vi "Sub_Preprocessing_Main.vi"(11 "Experiment in":T1) -> (3 "Experiment out":T1)   [LabVIEW 2021]
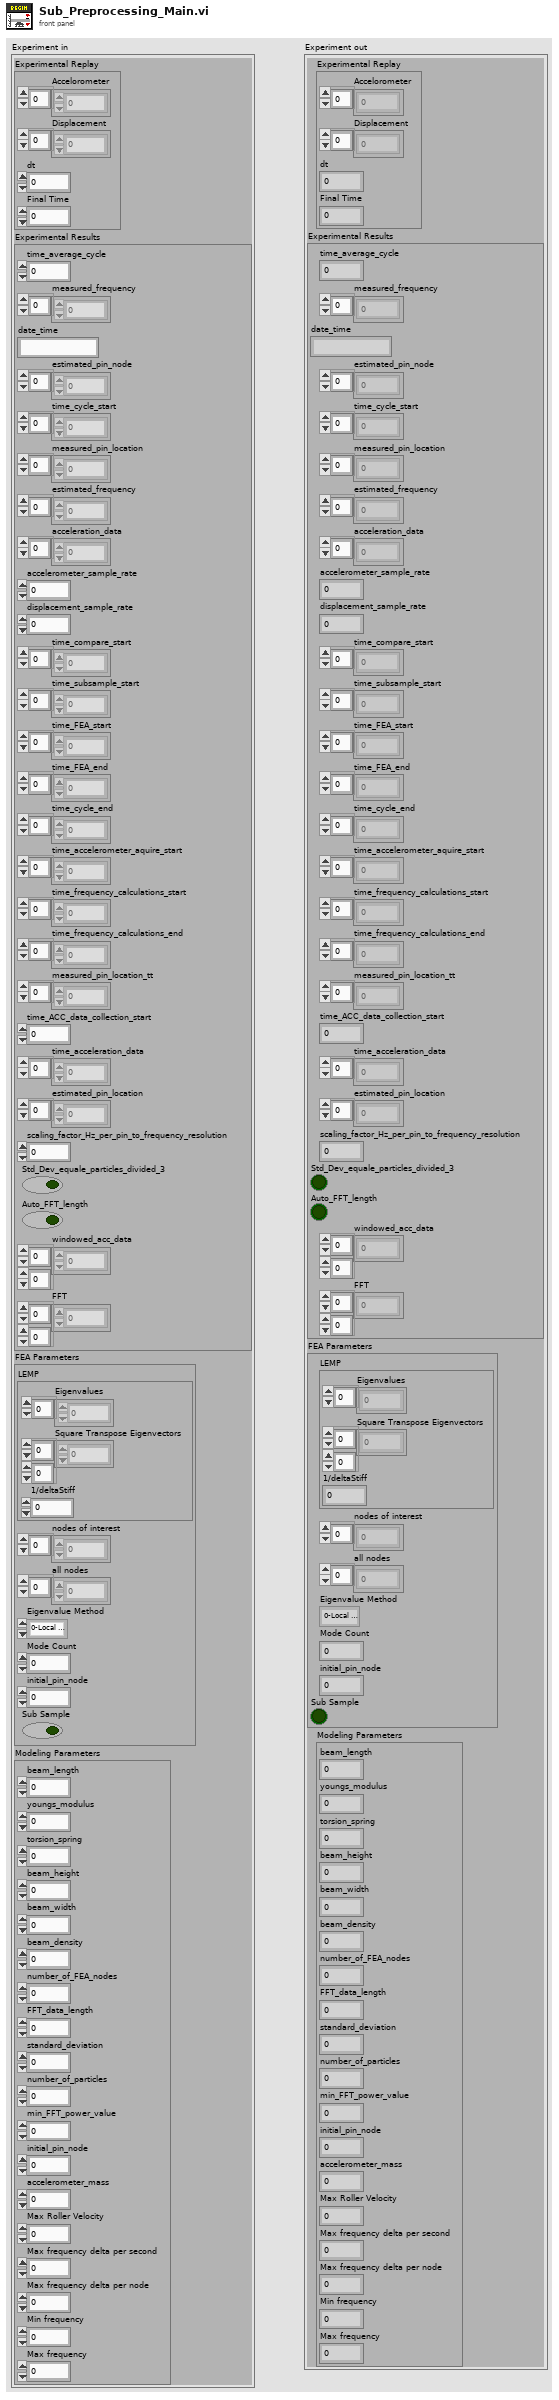
[diagram p1: front panel]
types:
  T1 = cluster{"Experimental Replay":cluster{"Accelorometer":dbl[], "Displacement":dbl[], "dt":dbl, "Final Time":dbl}, "Experimental Results":cluster{"time_average_cycle":dbl, "measured_frequency":dbl[], "date_time":string, "estimated_pin_node":i32[], "time_cycle_start":dbl[], "measured_pin_location":dbl[], "estimated_frequency":dbl[], "acceleration_data":dbl[], "accelerometer_sample_rate":dbl, "displacement_sample_rate":dbl, "time_compare_start":dbl[], "time_subsample_start":dbl[], "time_FEA_start":dbl[], "time_FEA_end":dbl[], "time_cycle_end":dbl[], "time_accelerometer_aquire_start":dbl[], "time_frequency_calculations_start":dbl[], "time_frequency_calculations_end":dbl[], "measured_pin_location_tt":dbl[], "time_ACC_data_collection_start":dbl, "time_acceleration_data":dbl[], "estimated_pin_location":dbl[], "scaling_factor_Hz_per_pin_to_frequency_resolution":dbl, "Std_Dev_equale_particles_divided_3":bool, "Auto_FFT_length":bool, "windowed_acc_data":dbl[][], "FFT":dbl[][]}, "FEA Parameters":cluster{"LEMP":cluster{"Eigenvalues":dbl[], "Square Transpose Eigenvectors":dbl[][], "1/deltaStiff":dbl}, "nodes of interest":i32[], "all nodes":i32[], "Eigenvalue Method":enum16{"0-Local Eigen Modification Procedure", "1-LabVIEW generalized eigenvalues", "2-LabVIEW M^-1K eigenvalues", "3-LabVIEW Cholesky Factorization", "4-Cholesky Factorization CPU SGL", "5-Cholesky Factorization CPU FXP", "6-Cholesky Factorization FPGA SGL", "7-Cholesky Factorization FPGA SGL SCL"}, "Mode Count":i32, "initial_pin_node":i32, "Sub Sample":bool}, "Modeling Parameters":cluster{"beam_length":dbl, "youngs_modulus":dbl, "torsion_spring":dbl, "beam_height":dbl, "beam_width":dbl, "beam_density":dbl, "number_of_FEA_nodes":i32, "FFT_data_length":i32, "standard_deviation":dbl, "number_of_particles":i32, "min_FFT_power_value":dbl, "initial_pin_node":i32, "accelerometer_mass":dbl, "Max Roller Velocity":dbl, "Max frequency delta per second":dbl, "Max frequency delta per node":dbl, "Min frequency":dbl, "Max frequency":dbl}}
  T2 = cluster{"Accelorometer":dbl[], "Displacement":dbl[], "dt":dbl, "Final Time":dbl}
  T3 = cluster{"beam_length":dbl, "youngs_modulus":dbl, "torsion_spring":dbl, "beam_height":dbl, "beam_width":dbl, "beam_density":dbl, "number_of_FEA_nodes":i32, "FFT_data_length":i32, "standard_deviation":dbl, "number_of_particles":i32, "min_FFT_power_value":dbl, "initial_pin_node":i32, "accelerometer_mass":dbl, "Max Roller Velocity":dbl, "Max frequency delta per second":dbl, "Max frequency delta per node":dbl, "Min frequency":dbl, "Max frequency":dbl}
  T4 = cluster{"time_average_cycle":dbl, "measured_frequency":dbl[], "date_time":string, "estimated_pin_node":i32[], "time_cycle_start":dbl[], "measured_pin_location":dbl[], "estimated_frequency":dbl[], "acceleration_data":dbl[], "accelerometer_sample_rate":dbl, "displacement_sample_rate":dbl, "time_compare_start":dbl[], "time_subsample_start":dbl[], "time_FEA_start":dbl[], "time_FEA_end":dbl[], "time_cycle_end":dbl[], "time_accelerometer_aquire_start":dbl[], "time_frequency_calculations_start":dbl[], "time_frequency_calculations_end":dbl[], "measured_pin_location_tt":dbl[], "time_ACC_data_collection_start":dbl, "time_acceleration_data":dbl[], "estimated_pin_location":dbl[], "scaling_factor_Hz_per_pin_to_frequency_resolution":dbl, "Std_Dev_equale_particles_divided_3":bool, "Auto_FFT_length":bool, "windowed_acc_data":dbl[][], "FFT":dbl[][]}
  T5 = cluster{"LEMP":cluster{"Eigenvalues":dbl[], "Square Transpose Eigenvectors":dbl[][], "1/deltaStiff":dbl}, "nodes of interest":i32[], "all nodes":i32[], "Eigenvalue Method":enum16{"0-Local Eigen Modification Procedure", "1-LabVIEW generalized eigenvalues", "2-LabVIEW M^-1K eigenvalues", "3-LabVIEW Cholesky Factorization", "4-Cholesky Factorization CPU SGL", "5-Cholesky Factorization CPU FXP", "6-Cholesky Factorization FPGA SGL", "7-Cholesky Factorization FPGA SGL SCL"}, "Mode Count":i32, "initial_pin_node":i32, "Sub Sample":bool}
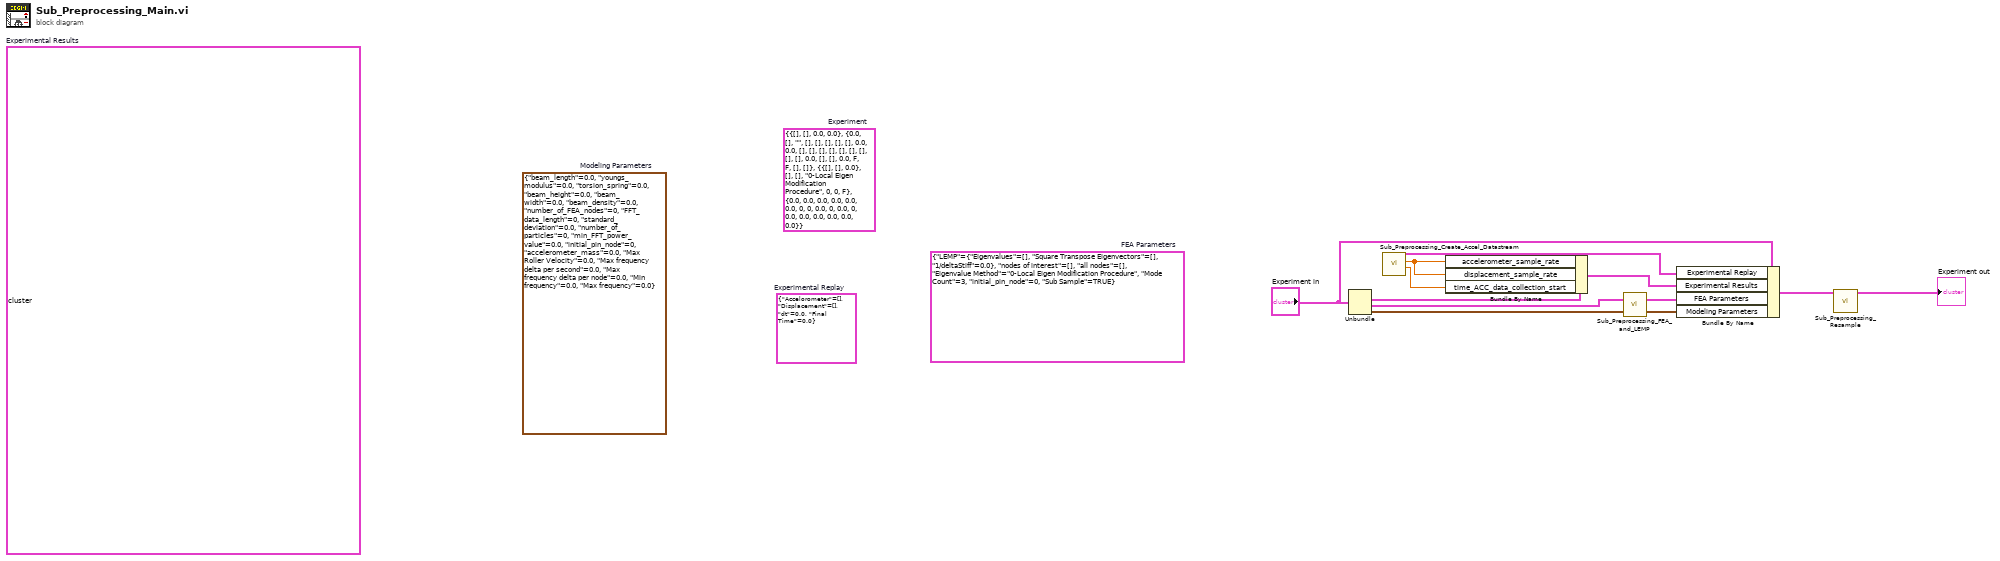
[diagram p0: block diagram]
diagram:
  (unwired) T1 {"Experimental Replay"={"Accelorometer"=[], "Displacement"=[], "dt"=0.0, "Final Time"=0.0}, "Experimental Results"={"time_average_cycle"=0.0, "measured_frequency"=[], "date_time"="", "estimated_pin_node"=[], "time_cycle_start"=[], "measured_pin_location"=[], "estimated_frequency"=[], "acceleration_data"=[], "accelerometer_sample_rate"=0.0, "displacement_sample_rate"=0.0, "time_compare_start"=[], "time_subsample_start"=[], "time_FEA_start"=[], "time_FEA_end"=[], "time_cycle_end"=[], "time_accelerometer_aquire_start"=[], "time_frequency_calculations_start"=[], "time_frequency_calculations_end"=[], "measured_pin_location_tt"=[], "time_ACC_data_collection_start"=0.0, "time_acceleration_data"=[], "estimated_pin_location"=[], "scaling_factor_Hz_per_pin_to_frequency_resolution"=0.0, "Std_Dev_equale_particles_divided_3"=FALSE, "Auto_FFT_length"=FALSE, "windowed_acc_data"=[], "FFT"=[]}, "FEA Parameters"={"LEMP"={"Eigenvalues"=[], "Square Transpose Eigenvectors"=[], "1/deltaStiff"=0.0}, "nodes of interest"=[], "all nodes"=[], "Eigenvalue Method"=enum."0-Local Eigen Modification Procedure", "Mode Count"=0, "initial_pin_node"=0, "Sub Sample"=FALSE}, "Modeling Parameters"={"beam_length"=0.0, "youngs_modulus"=0.0, "torsion_spring"=0.0, "beam_height"=0.0, "beam_width"=0.0, "beam_density"=0.0, "number_of_FEA_nodes"=0, "FFT_data_length"=0, "standard_deviation"=0.0, "number_of_particles"=0, "min_FFT_power_value"=0.0, "initial_pin_node"=0, "accelerometer_mass"=0.0, "Max Roller Velocity"=0.0, "Max frequency delta per second"=0.0, "Max frequency delta per node"=0.0, "Min frequency"=0.0, "Max frequency"=0.0}}  # Experiment
  (unwired) T2 {"Accelorometer"=[], "Displacement"=[], "dt"=0.0, "Final Time"=0.0}  # Experimental Replay
  (unwired) T3 {"beam_length"=0.0, "youngs_modulus"=0.0, "torsion_spring"=0.0, "beam_height"=0.0, "beam_width"=0.0, "beam_density"=0.0, "number_of_FEA_nodes"=0, "FFT_data_length"=0, "standard_deviation"=0.0, "number_of_particles"=0, "min_FFT_power_value"=0.0, "initial_pin_node"=0, "accelerometer_mass"=0.0, "Max Roller Velocity"=0.0, "Max frequency delta per second"=0.0, "Max frequency delta per node"=0.0, "Min frequency"=0.0, "Max frequency"=0.0}  # Modeling Parameters
  (unwired) T4 {"time_average_cycle"=0.0, "measured_frequency"=[], "date_time"="", "estimated_pin_node"=[], "time_cycle_start"=[], "measured_pin_location"=[], "estimated_frequency"=[], "acceleration_data"=[], "accelerometer_sample_rate"=0.0, "displacement_sample_rate"=0.0, "time_compare_start"=array[564 elements], "time_subsample_start"=array[564 elements], "time_FEA_start"=array[564 elements], "time_FEA_end"=array[564 elements], "time_cycle_end"=array[564 elements], "time_accelerometer_aquire_start"=array[564 elements], "time_frequency_calculations_start"=array[564 elements], "time_frequency_calculations_end"=array[564 elements], "measured_pin_location_tt"=array[564 elements], "time_ACC_data_collection_start"=0.0, "time_acceleration_data"=array[564 elements], "estimated_pin_location"=array[564 elements], "scaling_factor_Hz_per_pin_to_frequency_resolution"=1.0, "Std_Dev_equale_particles_divided_3"=TRUE, "Auto_FFT_length"=TRUE, "windowed_acc_data"=array1x564[564 elements], "FFT"=array1x564[564 elements]}  # Experimental Results
  (unwired) T5 {"LEMP"={"Eigenvalues"=[], "Square Transpose Eigenvectors"=[], "1/deltaStiff"=0.0}, "nodes of interest"=[], "all nodes"=[], "Eigenvalue Method"=enum."0-Local Eigen Modification Procedure", "Mode Count"=3, "initial_pin_node"=0, "Sub Sample"=TRUE}  # FEA Parameters
  n1 = Unbundle("Experiment in") -> ("Experimental Results"=w4:T4, "FEA Parameters"=w6:T5, "Modeling Parameters"=w5:T3)  [unwired: 1 out]
  n2 = call "Sub_Preprocessing_Create_Accel_Datastream.vi"() -> ("Start time"=w10:dbl, "Sample rate"=w11:dbl, "Experimental Replay"=w9:T2)  [unwired: 9 in]
  n3 = Bundle By Name(cluster=w4, "accelerometer_sample_rate"=w11, "displacement_sample_rate"=w11, "time_ACC_data_collection_start"=w10) -> (w12:T4)
  n4 = call "Sub_Preprocessing_FEA_and_LEMP.vi"("Modeling Parameters"=w5, "FEA Parameters"=w6) -> ("Modeling Parameters"=w8:T3, "FEA Parameters"=w7:T5)
  n5 = Bundle By Name(cluster="Experiment in", "Experimental Replay"=w9, "Experimental Results"=w12, "FEA Parameters"=w7, "Modeling Parameters"=w8) -> (w2:T1)
  n6 = call "Sub_Preprocessing_Resample.vi"("Experiment in"=w2) -> ("Experiment"=→"Experiment out":T1)  [unwired: 10 in]
